vi "PathPlanner_Cmd_FindPathPack.vi"(8 "Rotation Delay Distance M":dbl, 9 "Goal End Velocity M/S":dbl, 10 "PathPlannerPathConstraints":T4={"MaxVelocityMps;"=0.0, "MaxAccelerationMpsSq;"=0.0, "MaxAngularVelRadPsEc;"=0.0, "MaxAngularAccRadPSecSq"=0.0, "Exists"=FALSE, "Unlimited"=FALSE, "NominalVoltageVolts"=12.0}, 11 "Target Pose M":T1={"TRANSLATION"={"X"=0.0, "Y"=0.0}, "ROTATION"={"VALUE"=0.0, "COS"=1.0, "SIN"=0.0}} {"ROTATION"."SIN" format="%13.4f"; "ROTATION"."COS" format="%13.4f"; "ROTATION"."VALUE" format="%13.4f"; "TRANSLATION"."Y" format="%14.3f"; "TRANSLATION"."X" format="%14.3f"}) -> (3 "PathPlanner_Cmd_FindConfig":T5={"Goal Position"={"X"=0.0, "Y"=0.0}, "GoalEndState"={"VelocityMPS"=0.0, "Rotation"={"VALUE"=0.0, "COS"=1.0, "SIN"=0.0}}, "PathPlannerPathConstraints"={"MaxVelocityMps;"=0.0, "MaxAccelerationMpsSq;"=0.0, "MaxAngularVelRadPsEc;"=0.0, "MaxAngularAccRadPSecSq"=0.0, "Exists"=FALSE, "Unlimited"=FALSE, "NominalVoltageVolts"=12.0}, "Rotation Delay Distance M"=0.0} {"GoalEndState"."Rotation"."SIN" format="%13.4f"; "GoalEndState"."Rotation"."COS" format="%13.4f"; "GoalEndState"."Rotation"."VALUE" format="%13.4f"; "Goal Position"."Y" step=0.25 format="%14.3f"; "Goal Position"."X" format="%14.3f"})   [LabVIEW 2019, in "PathPlanner24.lvlib"]
doc: "DOCUMENTATION IS NOT COMPLETE.\n \nPack path finding configuration data.\n\nInputs:\n\nOutputs:"
uses:
  PathPlanner24.lvlib
  TypeDef/PathPlannerCmdFindConfig.ctl
  <vilib>/Rock Robotics/WPI/ThirdParty/JAS_Junk/TrajLib/TypeDef/TRANSLATION2D.ctl
  TypeDef/PathPlannerGoalEndState.ctl
  <vilib>/Rock Robotics/WPI/ThirdParty/JAS_Junk/TrajLib/TypeDef/ROTATION2D.ctl
  TypeDef/PathPlannerPathConstraints.ctl
  <vilib>/Rock Robotics/WPI/ThirdParty/JAS_Junk/TrajLib/TypeDef/POSE2D.ctl
  <vilib>/Rock Robotics/WPI/ThirdParty/JAS_Junk/TrajLib/Trajectory_Library.lvlib
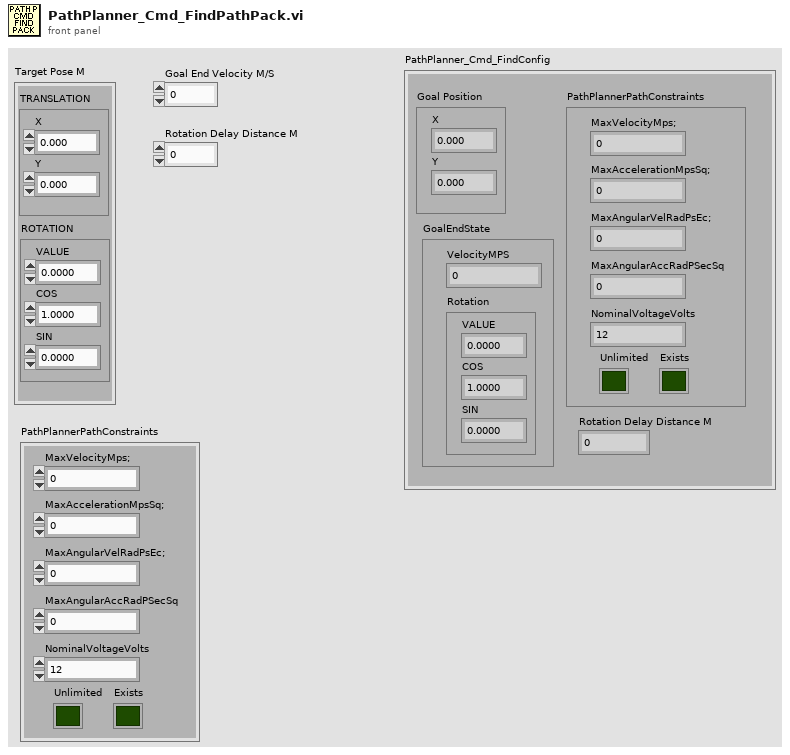
[diagram p1: front panel]
types:
  T1 = typedef "Trajectory_Library.lvlib/POSE2D.ctl" = cluster{"TRANSLATION":T2, "ROTATION":T3}
  T2 = typedef "Trajectory_Library.lvlib/TRANSLATION2D.ctl" = cluster{"X":dbl, "Y":dbl}
  T3 = typedef "Trajectory_Library.lvlib/ROTATION2D.ctl" = cluster{"VALUE":dbl, "COS":dbl, "SIN":dbl}
  T4 = typedef "PathPlanner24.lvlib/PathPlannerPathConstraints.ctl" = cluster{"MaxVelocityMps;":dbl, "MaxAccelerationMpsSq;":dbl, "MaxAngularVelRadPsEc;":dbl, "MaxAngularAccRadPSecSq":dbl, "Exists":bool, "Unlimited":bool, "NominalVoltageVolts":dbl}
  T5 = typedef "PathPlanner24.lvlib/PathPlannerCmdFindConfig.ctl" = cluster{"Goal Position":T2, "GoalEndState":T6, "PathPlannerPathConstraints":T4, "Rotation Delay Distance M":dbl}
  T6 = typedef "PathPlanner24.lvlib/PathPlannerGoalEndState.ctl" = cluster{"VelocityMPS":dbl, "Rotation":T3}
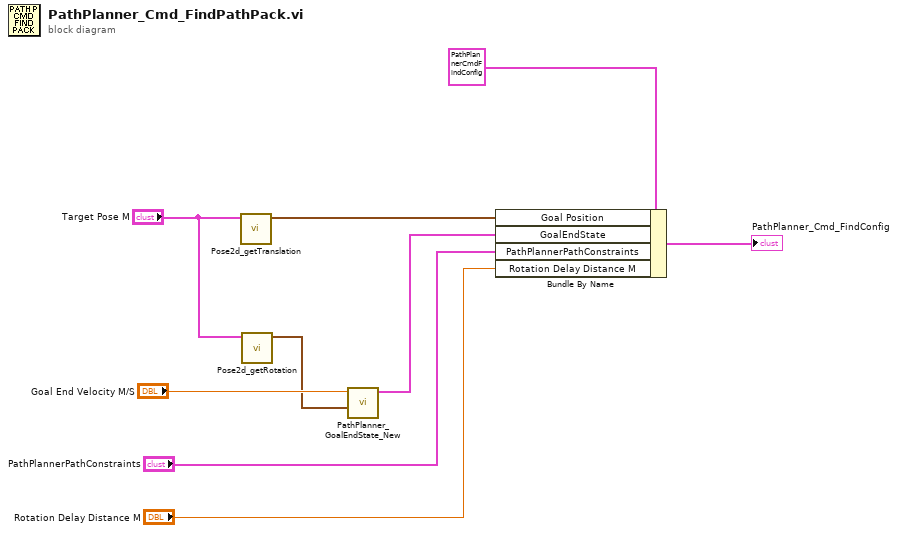
[diagram p0: block diagram]
diagram:
  n1 = call <vilib>:"Pose2d_getTranslation.vi"("in POSE"="Target Pose M") -> ("outTRANSLATION"=w4:T2)  [unwired: 10 in]
  n2 = call <vilib>:"Pose2d_getRotation.vi"("in POSE"="Target Pose M") -> ("out ROTATION"=w2:T3)  [unwired: 10 in]
  n3 = call "PathPlanner_GoalEndState_New.vi"("Rotation"=w2, "VelocityMPS"="Goal End Velocity M/S") -> ("GoalEndState"=w6:T6)  [unwired: 9 in]
  n4 = Bundle By Name(cluster=T5 {"Goal Position"={"X"=0.0, "Y"=0.0}, "GoalEndState"={"VelocityMPS"=0.0, "Rotation"={"VALUE"=0.0, "COS"=1.0, "SIN"=0.0}}, "PathPlannerPathConstraints"={"MaxVelocityMps;"=0.0, "MaxAccelerationMpsSq;"=0.0, "MaxAngularVelRadPsEc;"=0.0, "MaxAngularAccRadPSecSq"=0.0, "Exists"=FALSE, "Unlimited"=FALSE, "NominalVoltageVolts"=12.0}, "Rotation Delay Distance M"=0.0} ("PathPlanner_Cmd_FindConfig"), "Goal Position"=w4, "GoalEndState"=w6, "PathPlannerPathConstraints"="PathPlannerPathConstraints", "Rotation Delay Distance M"="Rotation Delay Distance M") -> (→"PathPlanner_Cmd_FindConfig":T5)
